vi "initialize creator.vi"(8 "error in":errorcluster, 10 "pointer":u64, 11 "connection creator in":refnum<class "connection creator.lvclass">) -> (0 "error out":errorcluster, 3 "connection creator out":refnum<class "connection creator.lvclass">)   [LabVIEW 2016, in "connection creator.lvclass"]
uses:
  connection creator.lvclass
  connection creator.lvclass/connection creator.ctl
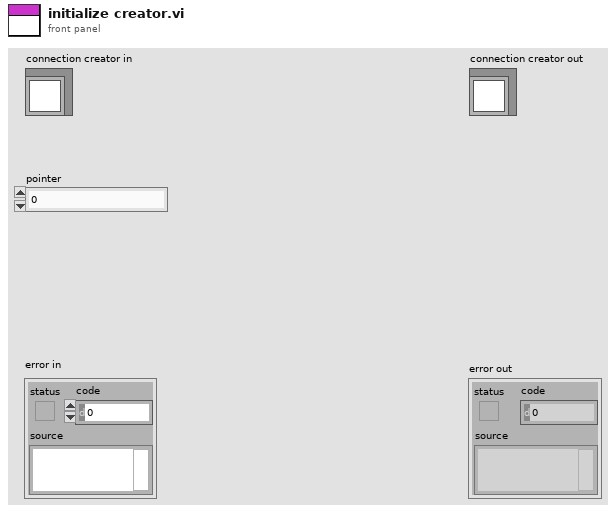
[diagram p1: front panel]
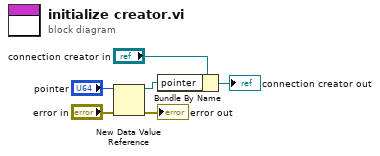
[diagram p0: block diagram]
diagram:
  n1 = New Data Value Reference(data value="pointer", error in="error in") -> (data value reference=w2:refnum<data-value>, error out=→"error out":errorcluster)
  n2 = Bundle By Name(cluster="connection creator in", "pointer"=w2) -> (→"connection creator out":refnum<class "connection creator.lvclass">)
